vi "N5765A_Initialize.vi"(8 "error in (no error)":errorcluster, 10 "Reset?":bool=TRUE, 11 "Resource name":string) -> (0 "error out":errorcluster, 3 "VISA resource name out":refnum<visa-resource-name>)   [LabVIEW 2015]
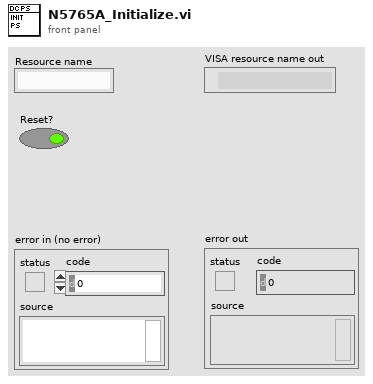
[diagram p1: front panel]
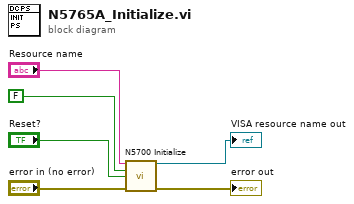
[diagram p0: block diagram]
diagram:
  n1 = call <instrlib>:"N5700 Initialize.vi"("VISA name"="Resource name", "ID Query (T)"=FALSE ("ID Query? (T: Yes)"), "Reset (T)"="Reset?", "error in (no error)"="error in (no error)") -> ("VISA out"=→"VISA resource name out":refnum<visa-resource-name>, "error out"=→"error out":errorcluster)  [unwired: 10 in]
